vi "QSM-PC Example.vi"() -> ()   [LabVIEW 2015]
uses:
  Resources/ctlSeqFNs.ctl
  Resources/ctlSeqFNs_SubVI 1.ctl
  Resources/ctlSeqFNs_SubVI 2.ctl
  <vilib>/Analysis/baseanly.llb/Mean (DBL).vi
  Resources/GLOBAL -MAIN.vi
  <vilib>/Analysis/NI_AALBase.lvlib
panel:
  out "deg C":dbl[](array[numeric])
  in  "STOP":bool
  in  "SendMsg":bool
  out "Date & Time":timestamp format="%<%.3X %x>T"
  out "Waveform Chart":dbl(graph)
  in  "Msg":string="<Type Message and Click Send>" caption="Type Message to Send to SubVI 1 and SubVI 2"
  # "Main Program"
  # "Recieves data from SubVI 2 and plots it"
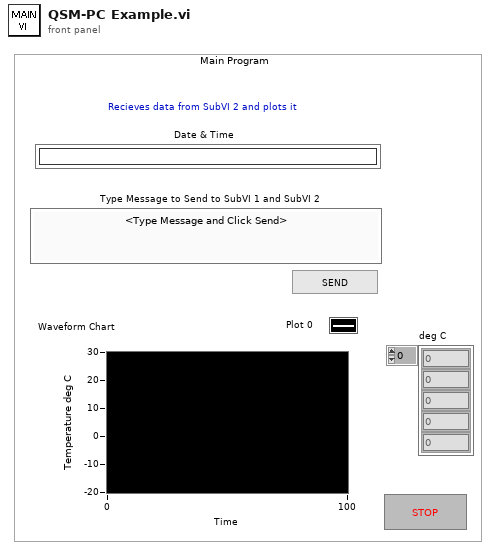
[diagram p1: front panel]
types:
  T1 = cluster{"VIRefNm":refnum<vi>, "CurrPath":path, "Results":cluster{"Kc":string, "Cfg":dbl[]}, "Q1":refnum<queue>, "Q2":refnum<queue>}
  T2 = typedef "ctlSeqFNs.ctl" = enum16{"INITIALIZE 00", "INITIALIZE 01", "IDLE", "Send Message to SubVIs", "PLOT RESULTS", "ERROR", "EXIT"}
  T3 = enum16{"ALIGN -CENTER", "ALIGN -TOP LEFT", "ALIGN -AS IS", "ALIGN -CUSTOM"}
  T4 = typedef "ctlSeqFNs_SubVI 2.ctl" = enum16{"INITIALIZE", "IDLE", "Convert deg F to deg C", "Send to Main", "Main Event Msg", "ERROR", "EXIT"}
  T5 = typedef "ctlSeqFNs_SubVI 1.ctl" = enum16{"INITIALIZE", "IDLE", "READ & SEND to SUBVI 2", "Main Event Msg", "ERROR", "EXIT"}
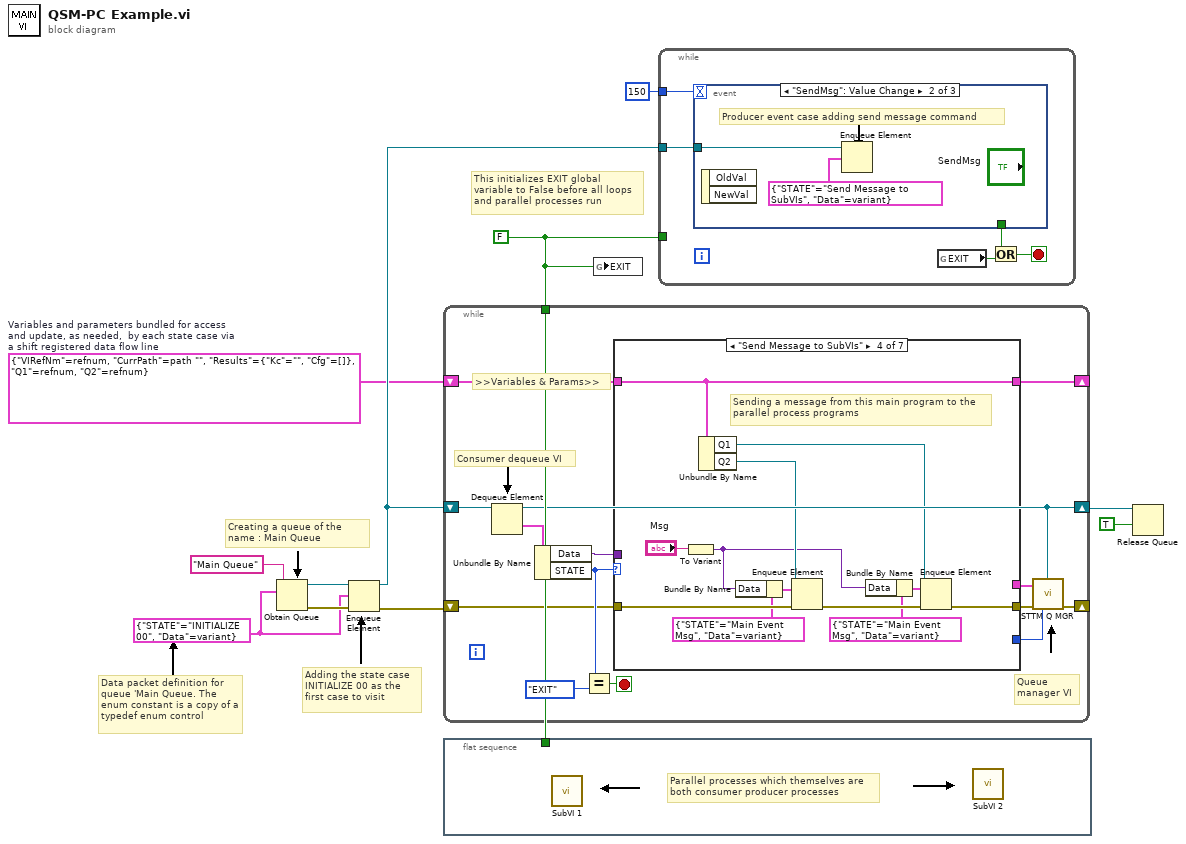
[diagram p0: block diagram]
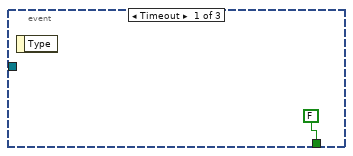
[diagram p2: hidden frame]
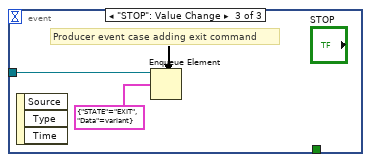
[diagram p3: hidden frame]
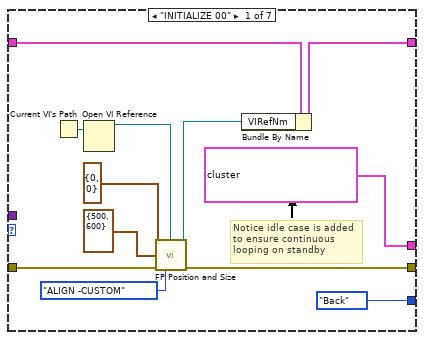
[diagram p4: hidden frame]
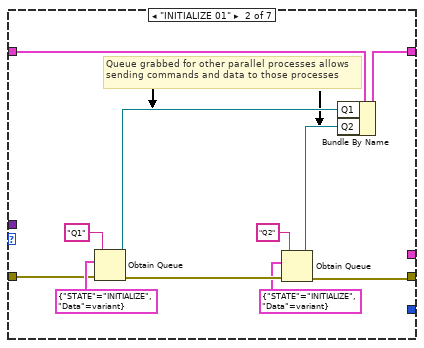
[diagram p5: hidden frame]
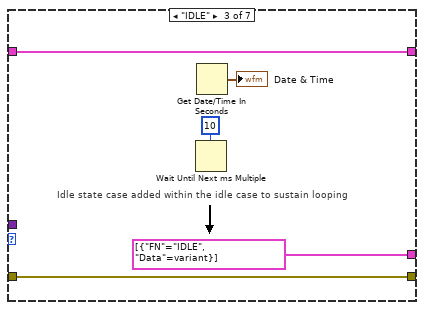
[diagram p6: hidden frame]
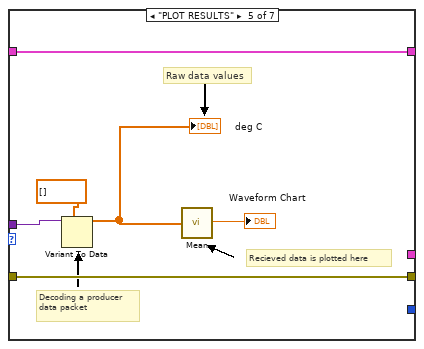
[diagram p7: hidden frame]
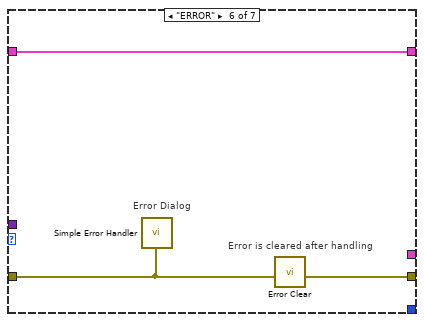
[diagram p8: hidden frame]
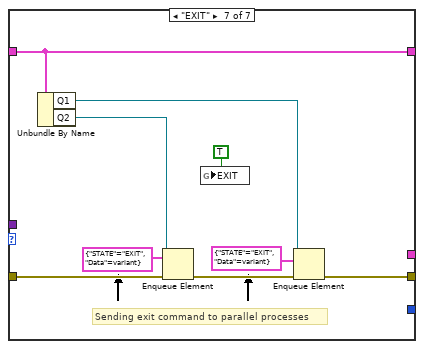
[diagram p9: hidden frame]
diagram:
  w2 = T1 {"VIRefNm"=refnum, "CurrPath"=path "", "Results"={"Kc"="", "Cfg"=[]}, "Q1"=refnum, "Q2"=refnum}  # Variables and parameters bundled for access and update, as needed,  by each state case via a shift registered data flow line
  w1 = FALSE
  w5 = cluster{"STATE":T2, "Data":variant} {"STATE"=enum."INITIALIZE 00", "Data"=variant} ("element")
  # "This initializes EXIT global variable to False before all loops and parallel processes run"
  # "Data packet definition for queue 'Main Queue. The enum constant is a copy of a typedef enum control"
  # "Adding the state case INITIALIZE 00 as the first case to visit"
  # "Creating a queue of the name : Main Queue"
  n1 = Obtain Queue(name (unnamed)="Main Queue" ("Queue Name"), element data type=w5) -> (queue out=w4:refnum<queue>, error out=w7:errorcluster)  [unwired: 3 in, 1 out]
  n2 = Enqueue Element(queue=w4, element=w5, error in (no error)=w7) -> (queue out=w3:refnum<queue>, error out=w6:errorcluster)  [unwired: 1 in, 1 out]
  n3 = while "State Machine" {
    shift-right: [w18] -> _
    shift-left: w6 -> [w16]
    shift-right: [w20] -> w9
    shift-left: w3 -> [w25]
    tunnel: w1 -> [_]
    shift-right: [w13] -> _
    shift-left: w2 -> [w14]
    stop <- w15 stop-if-true
    # "Queue manager VI"
    # "Consumer dequeue VI"
    # ">>Variables & Params>>"
    n4 = Dequeue Element(queue=w25) -> (queue out=w20:refnum<queue>, element=w24:cluster{"STATE":T2, "Data":variant})  [unwired: 2 in, 2 out]
    n5 = Unbundle By Name(w24) -> ("Data"=w23:variant, "STATE"=w22:T2)
    n6 = Equal?(x=w22, y=ctlSeqFNs."EXIT" ("FN")) -> (x = y?=w15:bool)
    n7 = case shown="\"Send Message to SubVIs\"" w22 {
      tunnel: w16 -> [w32 w38 w52 w65 w70 w73 w82]
      tunnel: [w31 w39 w52 w63 w70 w72 w80] -> w19
      tunnel: w23 -> [_ _ _ _ w69 _ _]
      tunnel: [cluster{"FN":T2, "Data":variant}[] [{"FN"=enum."INITIALIZE 01", "Data"=variant}, {"FN"=enum."IDLE", "Data"=variant}] _ cluster{"FN":T2, "Data":variant}[] [{"FN"=enum."IDLE", "Data"=variant}] _ _ _ _] -> w17
      tunnel: w14 -> [w30 w48 w53 w62 w71 w74 w79]
      tunnel: [w29 w47 w53 w62 w71 w74 w79] -> w13
      tunnel: [enum16{"Back", "Front", "Replace"}."Back" ("FNs") _ _ _ _ _ _] -> w12
      frame "INITIALIZE 00" {
        # "Notice idle case is added to ensure continuous looping on standby"
        n8 = Current VI's Path() -> (path=w33:path)
        n9 = Open VI Reference(vi path=w33) -> (vi reference=w34:refnum<vi>)  [unwired: 5 in, 1 out]
        n10 = call "FP Position and Size.vi"("VIRefNum  IN"=w34, "Poistion"=cluster{"left":i16, "top":i16} {"left"=0, "top"=0}, "Size"=cluster{"right":i16, "bottom":i16} {"right"=500, "bottom"=600}, "error in (no error)"=w32, "Mode"=T3."ALIGN -CUSTOM") -> ("VIRefNum OUT"=w28:refnum<vi>, "error out"=w31:errorcluster)  [unwired: 9 in]
        n11 = Bundle By Name(cluster=w30, "VIRefNm"=w28) -> (w29:T1)
      }
      frame "INITIALIZE 01" {
        # "Queue grabbed for other parallel processes allows sending commands and data to those processes"
        n12 = Obtain Queue(name (unnamed)="Q1", element data type=cluster{"STATE":T5, "Data":variant} {"STATE"=enum."INITIALIZE", "Data"=variant} ("element"), error in (no error)=w38) -> (queue out=w41:refnum<queue>, error out=w46:errorcluster)  [unwired: 2 in, 1 out]
        n13 = Obtain Queue(name (unnamed)="Q2", element data type=cluster{"STATE":T4, "Data":variant} {"STATE"=enum."INITIALIZE", "Data"=variant} ("element"), error in (no error)=w46) -> (queue out=w40:refnum<queue>, error out=w39:errorcluster)  [unwired: 2 in, 1 out]
        n14 = Bundle By Name(cluster=w48, "Q1"=w41, "Q2"=w40) -> (w47:T1)
      }
      frame "IDLE" {
        # "Idle state case added within the idle case to sustain looping"
        n15 = Wait Until Next ms Multiple(millisecond multiple=u32 10) -> ()  [unwired: 1 out]
        n16 = Get Date/Time In Seconds() -> (seconds since 1Jan1904=→"Date & Time":timestamp)
      }
      frame "Send Message to SubVIs" {
        # "Sending a message from this main program to the parallel process programs"
        n17 = To Variant(anything="Msg") -> (Variant=w57:variant)
        n18 = Unbundle By Name(w62) -> ("Q1"=w61:refnum<queue>, "Q2"=w60:refnum<queue>)
        n19 = Bundle By Name(cluster=cluster{"STATE":T4, "Data":variant} {"STATE"=enum."Main Event Msg", "Data"=variant} ("element"), "Data"=w57) -> (w55:cluster{"STATE":T4, "Data":variant})
        n20 = Enqueue Element(queue=w60, element=w55, error in (no error)=w65) -> (error out=w64:errorcluster)  [unwired: 1 in, 2 out]
        n21 = Bundle By Name(cluster=cluster{"STATE":T5, "Data":variant} {"STATE"=enum."Main Event Msg", "Data"=variant} ("element"), "Data"=w57) -> (w56:cluster{"STATE":T5, "Data":variant})
        n22 = Enqueue Element(queue=w61, element=w56, error in (no error)=w64) -> (error out=w63:errorcluster)  [unwired: 1 in, 2 out]
      }
      frame "PLOT RESULTS" {
        # "Raw data values"
        # "Recieved data is plotted here"
        # "Decoding a producer\ndata packet"
        n23 = Variant To Data(type=dbl[] [], Variant=w69) -> (data=w67:dbl[])  [unwired: 1 in, 1 out]
        "deg C" <- w67
        n24 = call-poly <vilib>:"Mean.vi"("X"=w67) -> ("mean"=→"Waveform Chart":dbl)  [unwired: 1 out]
      }
      frame "ERROR" {
        # "Error Dialog"
        # "Error is cleared after handling"
        n25 = call <vilib>:"Simple Error Handler.vi"("error in (no error)"=w73) -> ()  [unwired: 4 in, 5 out]
        n26 = call "Error Clear.vi"("error in"=w73) -> ("error in (no error)"=w72:errorcluster)  [unwired: 7 in]
      }
      frame "EXIT" {
        # "Sending exit command to parallel processes"
        n27 = Unbundle By Name(w79) -> ("Q1"=w78:refnum<queue>, "Q2"=w77:refnum<queue>)
        n28 = Enqueue Element(queue=w77, element=cluster{"STATE":T4, "Data":variant} {"STATE"=enum."EXIT", "Data"=variant}, error in (no error)=w82) -> (error out=w81:errorcluster)  [unwired: 1 in, 2 out]
        n29 = global write "GLOBAL -MAIN.vi" "EXIT"(TRUE ("EXIT")) -> ()
        n30 = Enqueue Element(queue=w78, element=cluster{"STATE":T5, "Data":variant} {"STATE"=enum."EXIT", "Data"=variant}, error in (no error)=w81) -> (error out=w80:errorcluster)  [unwired: 1 in, 2 out]
      }
    }
    n31 = call "STTM Q MGR.vi"("QSTATES"=w17, "QRef"=w20, "Error IN"=w19, "FNs"=w12) -> ("Error OUT"=w18:errorcluster)  [unwired: 11 in]
  }
  n32 = flat-sequence {
    tunnel: w1 -> [_]
    frame #0 {
      # "Parallel processes which themselves are both consumer producer processes"
      n33 = call "SubVI 1.vi"() -> ()  [unwired: 16 in]
      n34 = call "SubVI 2.vi"() -> ()  [unwired: 16 in]
    }
  }
  n35 = global write "GLOBAL -MAIN.vi" "EXIT"(w1) -> ()
  n36 = while "Events" {
    tunnel: 150 -> [w88]
    tunnel: w1 -> [_]
    tunnel: w3 -> [w84]
    stop <- w85 stop-if-true
    n37 = event shown="[1] \"SendMsg\": Value Change" {
      selector: _ -> [_ _ _]
      dyn-events: _ -> [_ _ _]
      timeout: w88 -> [_ _ _]
      tunnel: [FALSE _ _] -> w87
      tunnel: w84 -> [_ w91 w93]
      event Timeout {
        n38 = event-data() -> ()  [unwired: 1 in, 1 out]
      }
      event "SendMsg": Value Change {
        # "Producer event case adding send message command"
        n39 = event-data() -> ()  [unwired: 1 in, 2 out]
        n40 = Enqueue Element(queue=w91, element=cluster{"STATE":T2, "Data":variant} {"STATE"=enum."Send Message to SubVIs", "Data"=variant}) -> ()  [unwired: 2 in, 3 out]
      }
      event "STOP": Value Change {
        # "Producer event case adding exit command"
        n41 = event-data() -> ()  [unwired: 1 in, 3 out]
        n42 = Enqueue Element(queue=w93, element=cluster{"STATE":T2, "Data":variant} {"STATE"=enum."EXIT", "Data"=variant}) -> ()  [unwired: 2 in, 3 out]
      }
    }
    n43 = global read "GLOBAL -MAIN.vi" "EXIT"() -> (w86:bool)
    n44 = Or(x=w87, y=w86) -> (x .or. y?=w85:bool)
  }
  n45 = Release Queue(queue=w9, force destroy? (F)=TRUE) -> ()  [unwired: 1 in, 3 out]
